vi "Synchronize.vi"(7 "Retries (3)":i32=3, 8 "Error In":errorcluster, 11 "LINX Device Config":T1) -> (0 "Error Out":errorcluster, 3 "LINX Device Config":T1)   [LabVIEW 2020, in "LMH-LINX.lvlib" / "Device.lvlib"]
doc: "Synchronize the LINX device with LabVIEW."
uses:
  <vilib>/MakerHub/LINX/Private/Device/Device.lvlib
  <vilib>/MakerHub/LINX/LMH-LINX.lvlib
  <vilib>/MakerHub/LINX/Private/Type Defs/Error Type.ctl
  <vilib>/MakerHub/LINX/Private/Type Defs/Interface.ctl
  <vilib>/MakerHub/LINX/Private/Device/Type Defs/TCP Config.ctl
  <vilib>/MakerHub/LINX/Private/Device/Type Defs/LINX Device Config.ctl
  <vilib>/MakerHub/LINX/Private/Device/Type Defs/Channels.ctl
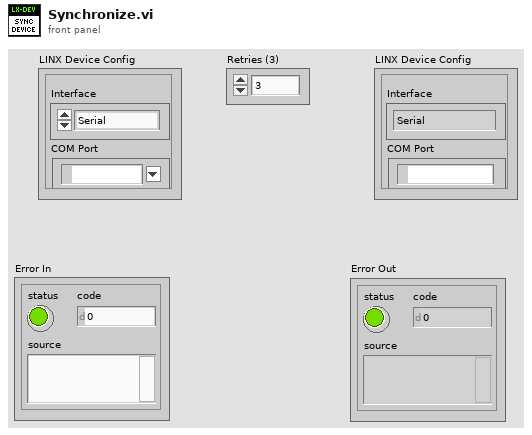
[diagram p1: front panel]
types:
  T1 = typedef "LMH-LINX.lvlib/Device.lvlib/LINX Device Config.ctl" = cluster{"Interface":T2, "COM Port":refnum<visa-resource-name>, "TCP Configuration":T3, "Device Family":u8, "Device ID":u8, "Device Name":string, "TCP Ref":refnum<k5>, "Channels":T4}
  T2 = typedef "LMH-LINX.lvlib/Interface.ctl" = enum16{"Serial", "TCP"}
  T3 = typedef "LMH-LINX.lvlib/Device.lvlib/TCP Config.ctl" = cluster{"IP Address":string, "Port":u16}
  T4 = typedef "LMH-LINX.lvlib/Channels.ctl" = cluster{"DI":u8[], "DO":u8[], "AI":u8[], "AO":u8[], "PWM":u8[], "QE":u8[], "UART":u8[], "I2C 2":u8[], "SPI":u8[], "CAN":u8[], "Servo":u8[], "AI Ref (V)":dbl, "AI Resolution (Bits)":u8, "AO Ref (V)":dbl, "AO Resolution (Bits)":u8}
  T5 = typedef "LMH-LINX.lvlib/Error Type.ctl" = enum16{"Unknown", "Timeout", "Corrupt Return Packet", "Unable To Connect", "Command Not Supported", "Channel DNE", "Invalid COM Config", "Firmware Version Mismatch", "myRIO Support", "CMD Specific Error", "Local IO Not Supported"}
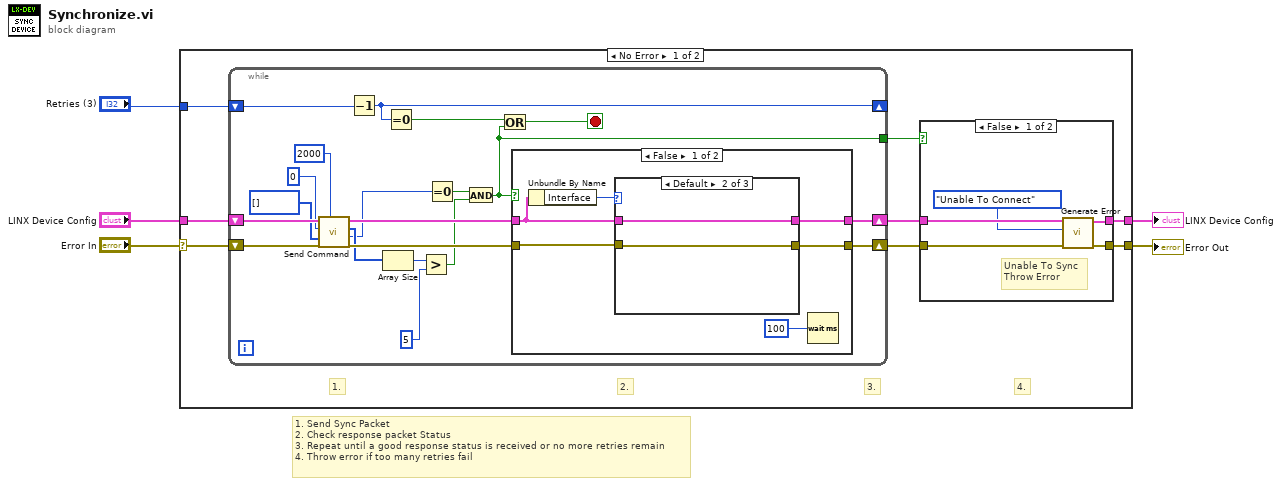
[diagram p0: block diagram]
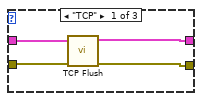
[diagram p3: hidden frame]
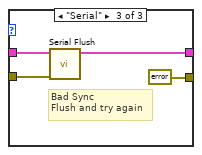
[diagram p4: hidden frame]
diagram:
  # "1. Send Sync Packet\n2. Check response packet Status\n3. Repeat until a good response status is received or no more retries remain\n4. Throw error if too many retries fail"
  n1 = case shown="No Error" "Error In" {
    selector: "Error In" -> [w6 w60]
    tunnel: "Retries (3)" -> [w13 _]
    tunnel: "LINX Device Config" -> [w12 w59]
    tunnel: [w8 w59] -> w3
    tunnel: [w7 w60] -> w2
    frame No Error {
      # "4."
      # "3."
      # "2."
      # "1."
      n2 = while {
        shift-right: [w35] -> _
        shift-left: w13 -> [w36]
        shift-right: [w31] -> w10
        shift-left: w6 -> [w39]
        tunnel: [w23] -> w9
        shift-right: [w33] -> w11
        shift-left: w12 -> [w40]
        stop <- w29 stop-if-true
        n3 = call <vilib>:"Send Command.vi"("Timeout (100 ms)"=2000, "Error In"=w39, "ARGS"=u8[] [], "CMD"=u16 0, "LINX Device Config"=w40) -> ("Error Out"=w30:errorcluster, "Status"=w22:u8, "Response"=w28:u8[], "LINX Device Config"=w32:T1)  [unwired: 3 in]
        n4 = Decrement(x=w36) -> (x-1=w35:i32)
        n5 = Array Size(array=w28) -> (size(s)=w27:i32)
        n6 = Equal To 0?(x=w35) -> (x = 0?=w34:bool)
        n7 = Greater?(x=w27, y=5) -> (0:w25:bool)
        n8 = Equal To 0?(x=w22) -> (x = 0?=w24:bool)
        n9 = And(x=w24, y=w25) -> (x .and. y?=w23:bool)
        n10 = Or(x=w34, y=w23) -> (x .or. y?=w29:bool)
        n11 = case shown="False" w23 {
          tunnel: [w44 w58] -> w33
          tunnel: w32 -> [w43 w58]
          tunnel: [w41 w57] -> w31
          tunnel: w30 -> [w46 w57]
          frame False {
            n12 = Unbundle By Name(w43) -> ("Interface"=w42:T2)
            n13 = case shown="Default" w42 {
              tunnel: w43 -> [w50 w52 w56]
              tunnel: w46 -> [w47 w51 w55]
              tunnel: [w49 w52 w54] -> w44
              tunnel: [w48 w51 errorcluster {"status"=FALSE, "code"=0, "source"=""} ("Error Out")] -> w41
              frame "TCP" {
                n14 = call <vilib>:"TCP Flush.vi"("Error In"=w47, "LINX Device Config"=w50) -> ("Error Out"=w48:errorcluster, "LINX Device Config"=w49:T1)  [unwired: 7 in, 1 out]
              }
              frame Default {
              }
              frame "Serial" {
                # "Bad Sync\nFlush and try again"
                n15 = call <vilib>:"Serial Flush.vi"("Error In"=w55, "LINX Device Config"=w56) -> ("LINX Device Config"=w54:T1)  [unwired: 8 in, 1 out]
              }
            }
            n16 = Wait (ms)(milliseconds to wait=u32 100) -> ()  [unwired: 1 out]
          }
          frame True {
            # "Sync OK"
          }
        }
      }
      n17 = case shown="False" w9 {
        tunnel: [w18 w20] -> w8
        tunnel: w11 -> [w16 w20]
        tunnel: [w17 w19] -> w7
        tunnel: w10 -> [w14 w19]
        frame False {
          # "Unable To Sync\nThrow Error"
          n18 = call <vilib>:"Generate Error.vi"("Error In"=w14, "Error Type"=Error_Type."Unable To Connect", "LINX Device Config"=w16) -> ("Error Out"=w17:errorcluster, "Dup LINX Device Config"=w18:T1)  [unwired: 7 in]
        }
        frame True {
          # "Sync OK"
        }
      }
    }
    frame Error {
    }
  }
  "Error Out" <- w2
  "LINX Device Config" <- w3
